vi "Waveform and Laser Controls V6.vi"() -> ()   [LabVIEW 2016]
uses:
  <vilib>/rvi/DataTransferAndStorage/Container/XNode/niFpgaContainer.xnode
  <vilib>/rvi/Memory/Memory_Emulation/nirvimemoryEmulation.vi
  <vilib>/rvi/Memory/Memory_Emulation/nirvimemoryFastEmulation.vi
  <vilib>/eio/EIONode/EIONode.xnode
  <vilib>/rvi/eio/common/nirviEmuTemplateMethod_errors.vi
  <vilib>/Platform/TimedLoop/XDataNode/wakeup.ctl
  <vilib>/Platform/TimedLoop/XDataNode/XDNodeRunTimeDep.lvlib
  <vilib>/Platform/TimedLoop/XDataNode/nitl_modes.ctl
  <vilib>/Platform/TimedLoop/XDataNode/timing_clust.ctl
  <vilib>/Platform/TimedLoop/XDataNode/XDataNode.xnode
  Waveform Scan Parameters.ctl
panel:
  out "Image Done?":bool
  in  "775 AOM (I16)":i16=16500
  in  "590 Analog Voltage (I16)":i16
  out "Laser Blank Trigger":bool
  in  "Laser On Time (Ticks)":u8=8
  in  "Sequences":u8=4
  in  "Laser Delay (Ticks)":u8
  in  "Laser States":u32
  in  "Blanking Off/Manual":bool
  in  "Z Piezo Axis":i16
  in  "Y Piezo Axis":i16
  in  "X Piezo Axis":i16
  out "End Linear Ramp":bool
  in  "End of Linear Ramp":u32
  in  "Z Stack Start Position (I16)":i16
  in  "Frames Per Z Step":u8
  in  "Number of Z Steps":u8
  in  "Z Step Size (I16)":i16
  in  "Stop Sync Signal":bool
  in  "Accums Per Line":u32[](array[numeric])=[0, 0, 0, 0]
  in  "Number of Lines":u32
  out "Frame Trigger":bool
  in  "Reset Position Error":bool
  in  "Galvo 1 Position (I16)":i16
  in  "Galvo 2 Position (I16)":i16
  in  "WF 3 Data Loaded":bool
  in  "WF 2 Data Loaded":bool
  in  "Waveform Scan Parameters":T1={"Scanning Mode"=0, "Fast Axis WF Length (Elements)"=0, "Fast Axis Sample Period (Ticks)"=40, "Slow Axis 1 WF Length (Elements)"=0, "Slow Axis 1 Sample Period (Ticks)"=40, "Slow Axis 1 Delay (25 ns) Steps"=40, "Slow Axis 2 WFLength (Elements)"=0, "Slow Axis 2 Sample Period (Ticks)"=40, "Slow Axis 2 Delay (25 ns) Steps"=40}
  in  "Resonant Mirror":T2
  in  "Galvo Mirror 2":T3
  in  "Galvo Mirror 1":T3
  in  "Start Waveforms":bool
  in  "Unused Axis Offset":i16
  in  "Slow Axis 2 Waveform Element":i16
  in  "Fast Axis Waveform Element":i16
  in  "Slow Axis 1 Waveform Element":i16
  in  "WF 1 Data Loaded":bool
  # "Copyright (C) 2020 Edward S Allgeyer\n\nRedistribution and use in source and binary forms, with or without\nmodification, are permitted provided that the following conditions\nare met:\n\n1. Redistributions of source code must retain the above copyright\n   notice, this list of conditions and the following disclaimer.\n\n2. Redistributions in binary form must reproduce the above copyright\n   notice, this list of conditions and the following disclaimer in\n   the documentation and/or other materials provided with the\n   distribution.\n\n3. Neither the name of the copyright holder nor the names of its\n   contributors may be used to endorse or promote products derived\n   from this software without specific prior written permission.\n\nTHIS SOFTWARE IS PROVIDED BY THE COPYRIGHT HOLDERS AND CONTRIBUTORS\n\"AS IS\" AND ANY EXPRESS OR IMPLIED WARRANTIES, INCLUDING, BUT NOT\nLIMITED TO, THE IMPLIED WARRANTIES OF MERCHANTABILITY AND FITNESS\nFOR A PARTICULAR PURPOSE ARE DISCLAIMED. IN NO EVENT SHALL THE\nCOPYRIGHT HOLDER OR CONTRIBUTORS BE LIABLE FOR ANY DIRECT, INDIRECT,\nINCIDENTAL, SPECIAL, EXEMPLARY, OR CONSEQUENTIAL DAMAGES (INCLUDING,\nBUT NOT LIMITED TO, PROCUREMENT OF SUBSTITUTE GOODS OR SERVICES;\nLOSS OF USE, DATA, OR PROFITS; OR BUSINESS INTERRUPTION) HOWEVER\nCAUSED AND ON ANY THEORY OF LIABILITY, WHETHER IN CONTRACT, STRICT\nLIABILITY, OR TORT (INCLUDING NEGLIGENCE OR OTHERWISE) ARISING IN\nANY WAY OUT OF THE USE OF THIS SOFTWARE, EVEN IF ADVISED OF THE\nPOSSIBILITY OF SUCH DAMAGE."
  # "V2 - Adding in a line clock\nV3 - Cluster Scan Parameters"
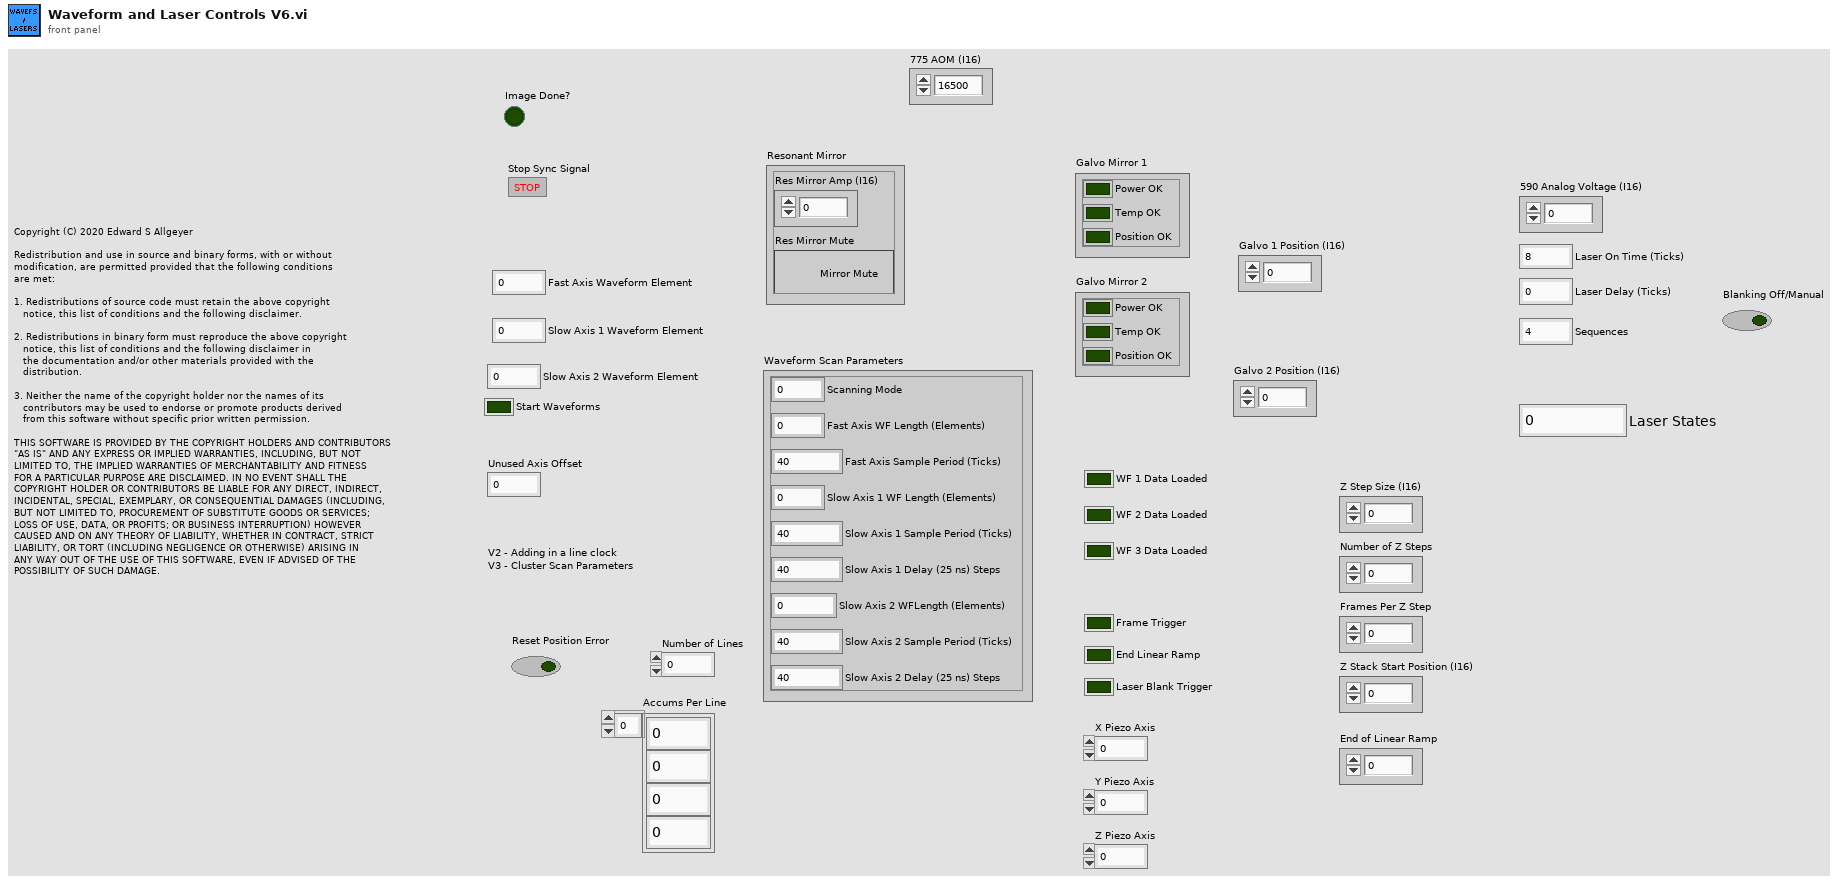
[diagram p1: front panel]
types:
  T1 = typedef "Waveform Scan Parameters.ctl" = cluster{"Scanning Mode":u8, "Fast Axis WF Length (Elements)":i32, "Fast Axis Sample Period (Ticks)":u32, "Slow Axis 1 WF Length (Elements)":i32, "Slow Axis 1 Sample Period (Ticks)":u32, "Slow Axis 1 Delay (25 ns) Steps":i32, "Slow Axis 2 WFLength (Elements)":i32, "Slow Axis 2 Sample Period (Ticks)":u32, "Slow Axis 2 Delay (25 ns) Steps":i32}
  T2 = cluster{"Res Mirror Amp (I16)":i16, "Res Mirror Mute":bool}
  T3 = cluster{"Power OK":bool, "Temp OK":bool, "Position OK":bool}
  T4 = typedef "XDNodeRunTimeDep.lvlib/timing_clust.ctl" = cluster{"Expected End [f-1]":u64, "Actual End [f-1]":u64, "Finished Late? [f-1]":bool, "Expected End [i-1]":u64, "Actual End [i-1]":u64, "Finished Late? [i-1]":bool, "Expected Start [i]":u64, "Actual Start [i]":u64, "Expected Start [f]":u64, "Actual Start [f]":u64, "Source Name":string, "Structure Name":string, "Period":i64, "Deadline":i64, "Offset":i64, "Start":i64, "Priority":i32, "Timeout":i32, "Mode":T5, "Wakeup Reason":T6, "Error":errorcluster, "Source Type":string, "Secondary Source Type":string, "Global End Time":u64, "Global Start Time":u64, "Frame Duration":u64, "Iteration Duration":u64, "Assigned CPU":i32, "I/O Scan Engine Mode":u32}
  T5 = typedef "XDNodeRunTimeDep.lvlib/nitl_modes.ctl" = enum32{"No Change", "Process missed periods, maintain original phase", "Discard missed periods, maintain original phase", "Process missed periods, ignore original phase", "Discard missed periods, ignore original phase"}
  T6 = typedef "XDNodeRunTimeDep.lvlib/wakeup.ctl" = enum32{"Normal", "Aborted", "Asynchronous wakeup", "Timing source error", "Timed loop error", "Timeout"}
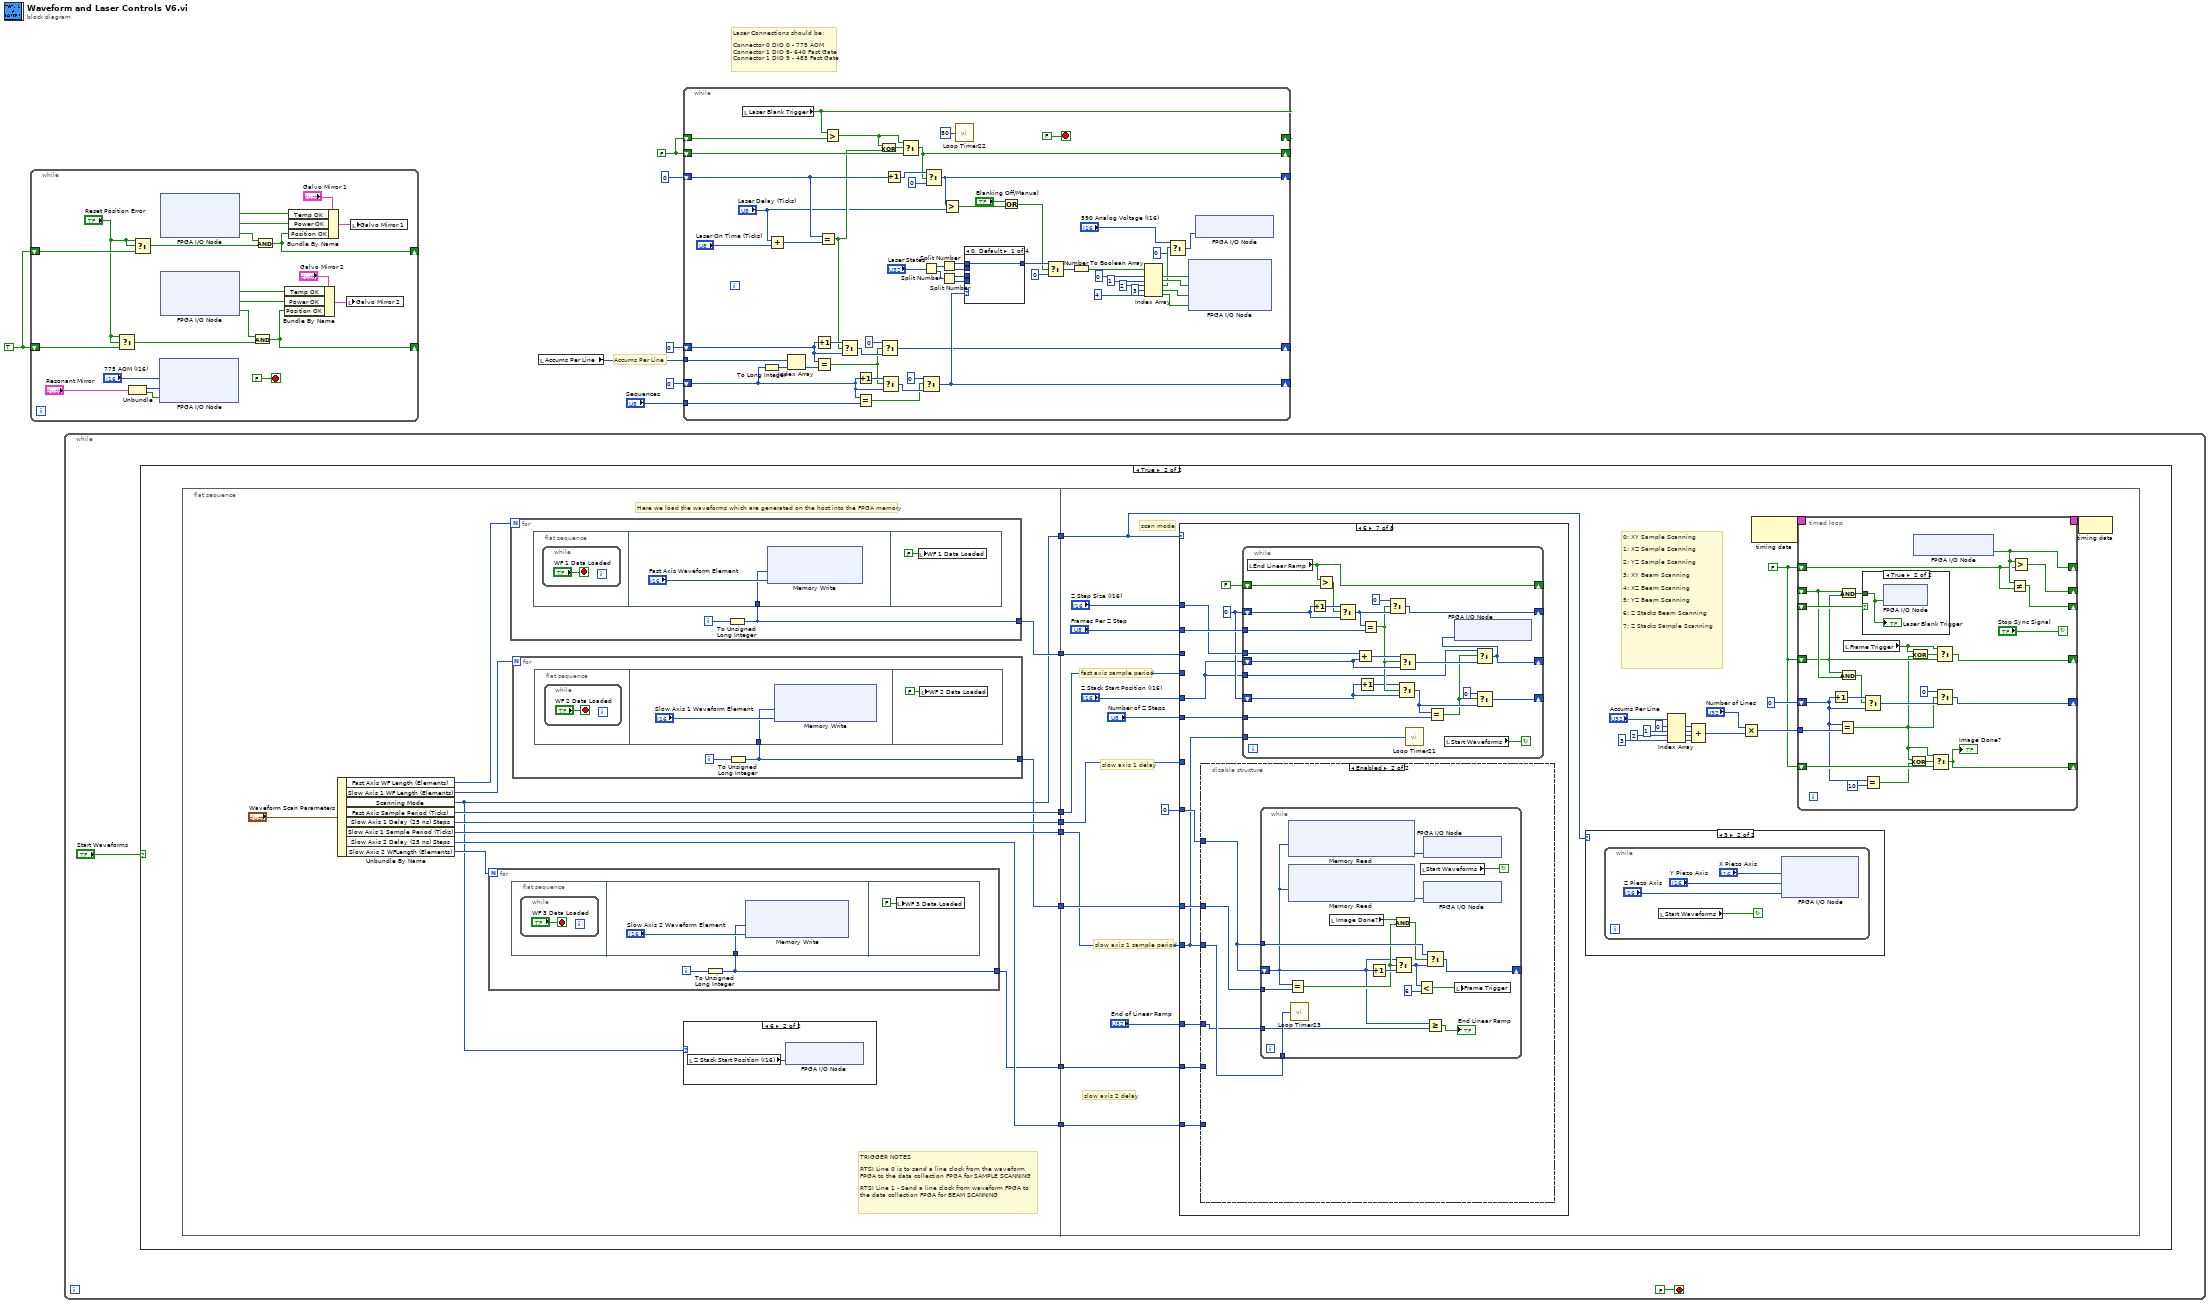
[diagram p0: block diagram]
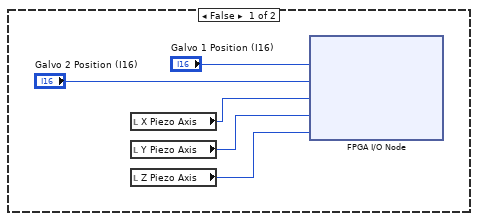
[diagram p5: hidden frame]
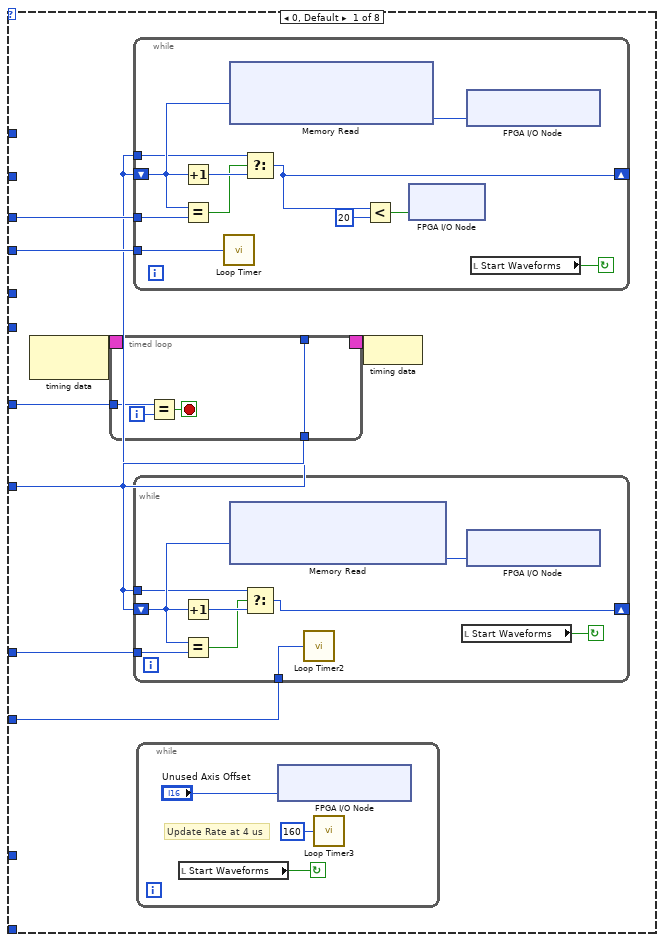
[diagram p9: hidden frame]
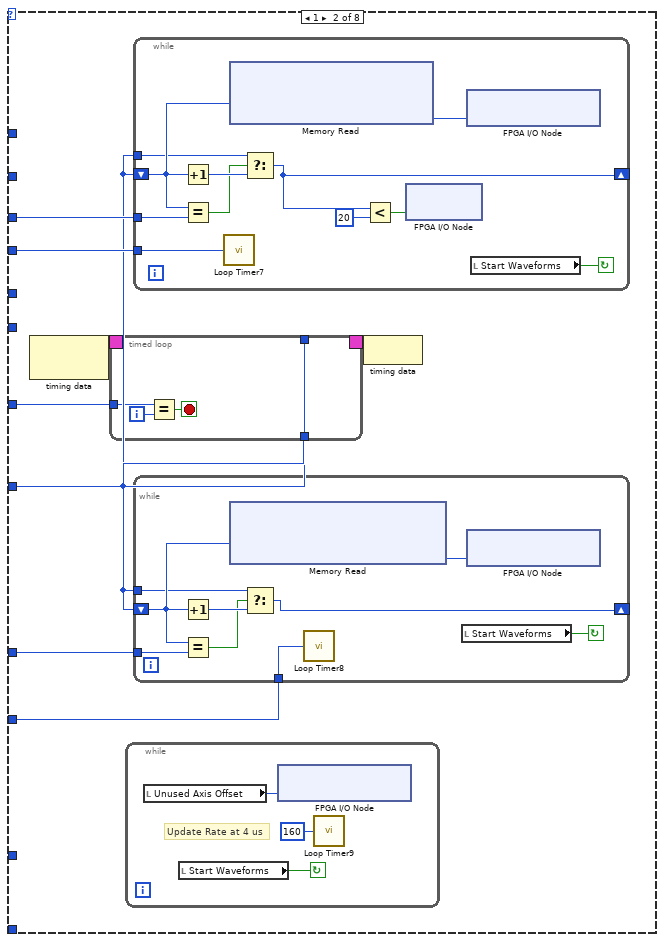
[diagram p10: hidden frame]
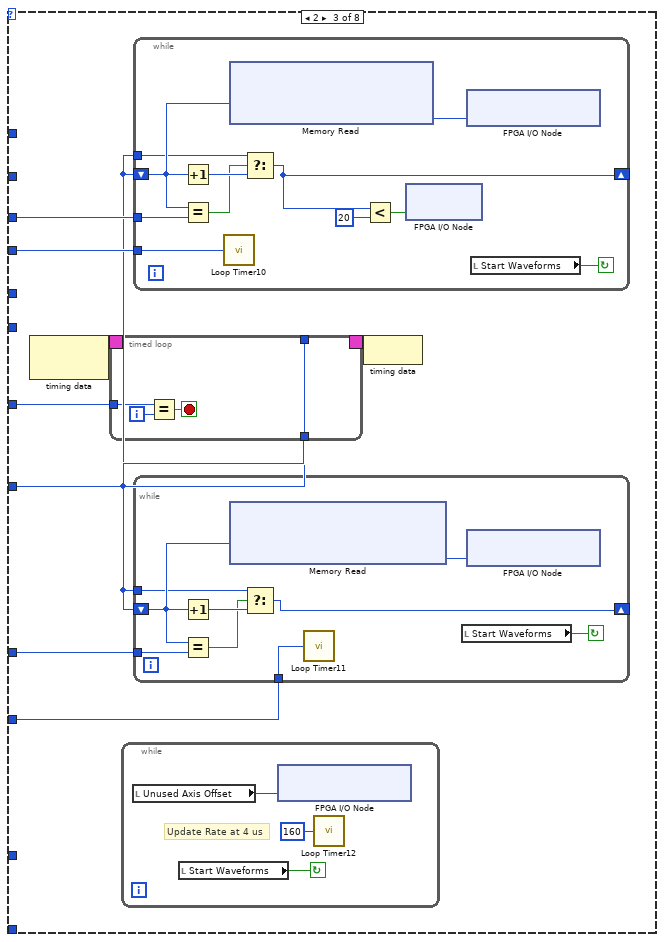
[diagram p11: hidden frame]
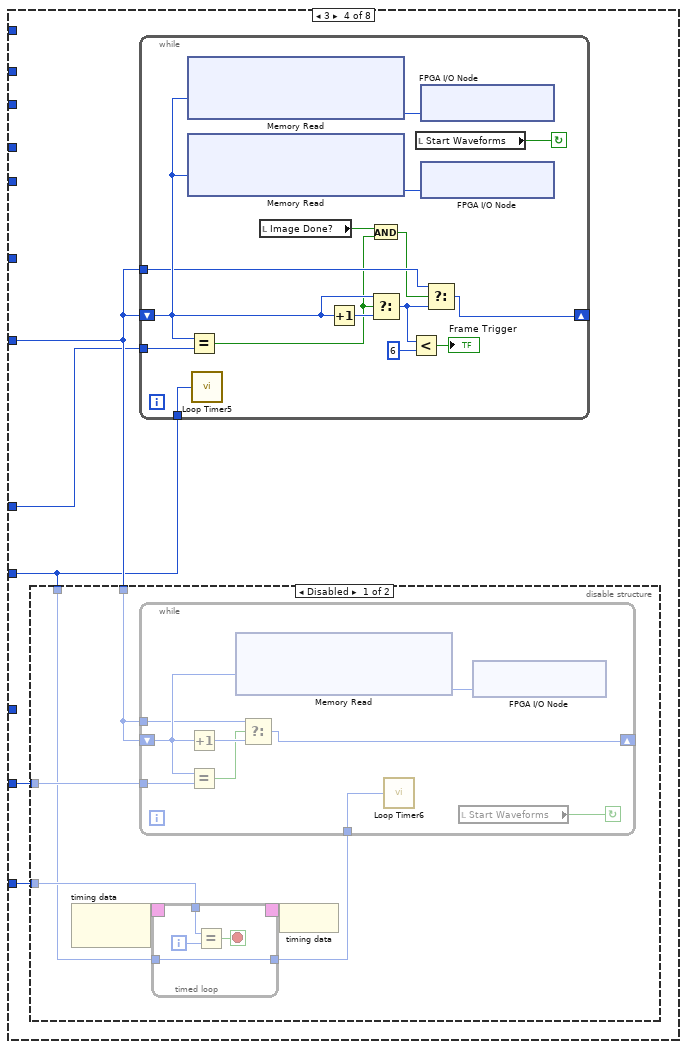
[diagram p12: hidden frame]
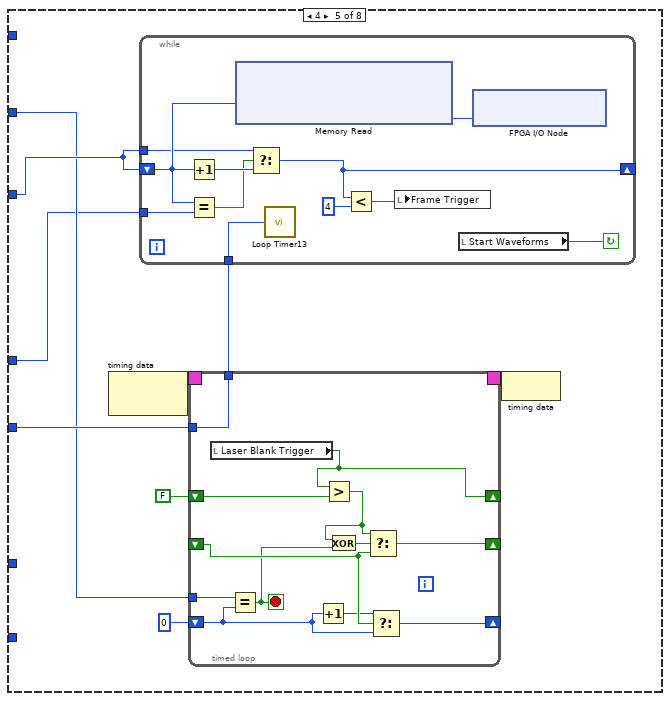
[diagram p14: hidden frame]
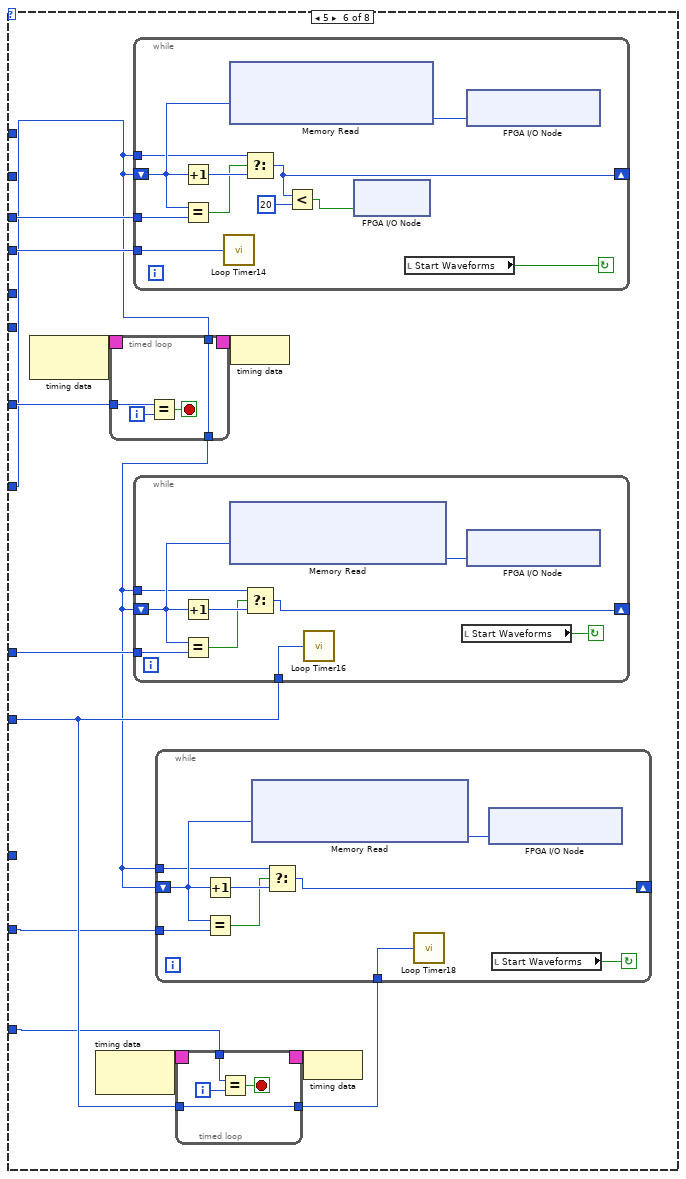
[diagram p15: hidden frame]
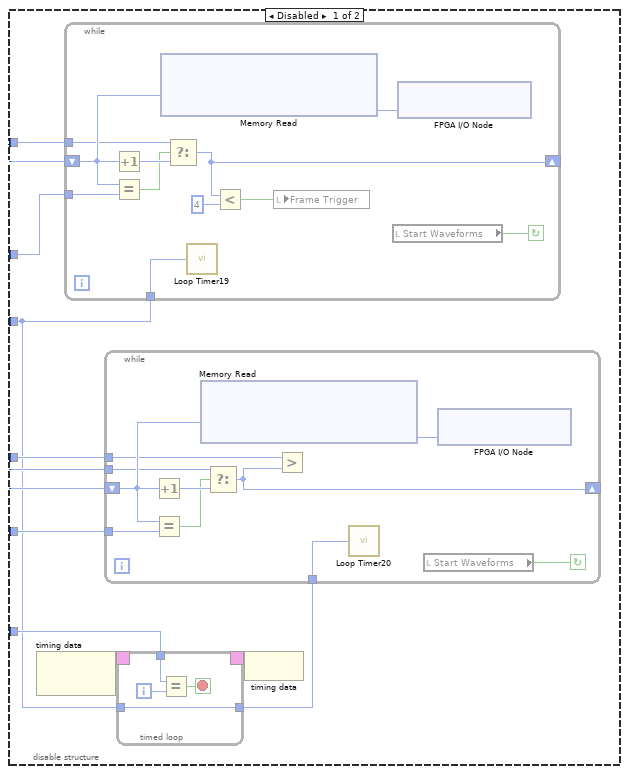
[diagram p16: hidden frame]
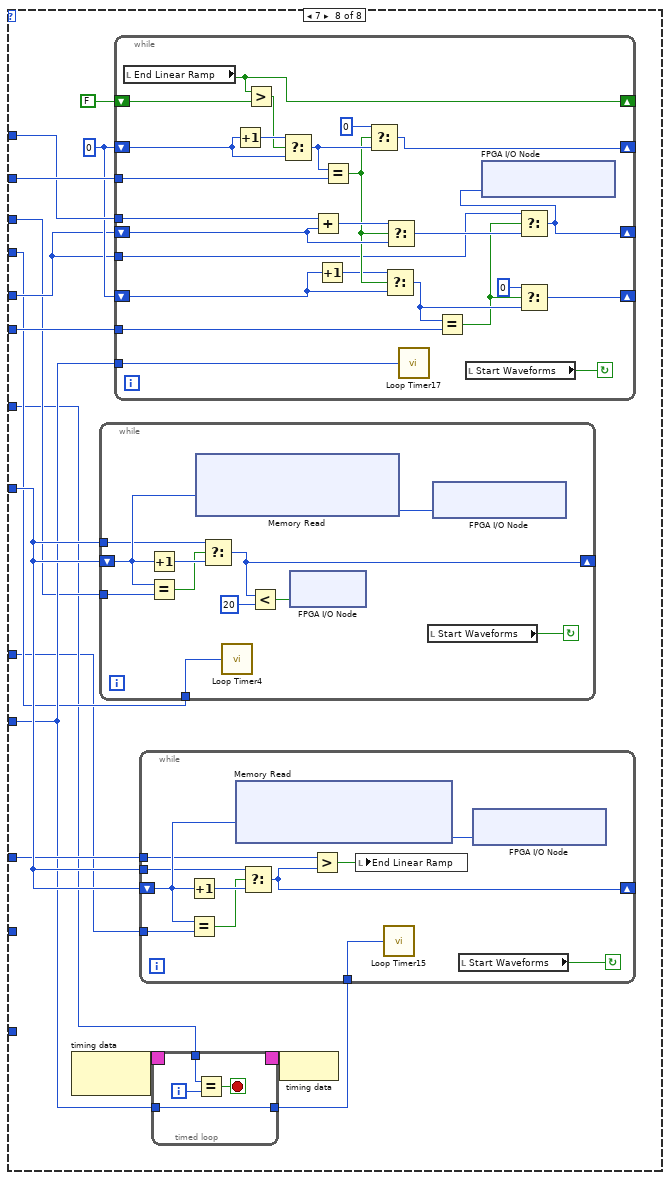
[diagram p17: hidden frame]
diagram:
  w2 = FALSE
  w7 = TRUE
  # "Laser Connections should be:\n\nConnector 0 DIO 0 - 775 AOM\nConnector 1 DIO 8- 640 Fast Gate\nConnector 1 DIO 9 - 485 Fast Gate"
  # "Accums Per Line"
  n1 = while {
    shift-right: [w14] -> _
    shift-left: w7 -> [w16]
    shift-right: [w10] -> _
    shift-left: w7 -> [w12]
    stop <- FALSE stop-if-true
    n2 = Select(t="Reset Position Error", s="Reset Position Error", f=w16) -> (s? t:f=w15:bool)
    n3 = Unbundle("Resonant Mirror") -> ("Res Mirror Amp (I16)"=w27:i16, "Res Mirror Mute"=w26:bool)
    n4 = Select(t="Reset Position Error", s="Reset Position Error", f=w12) -> (s? t:f=w11:bool)
    n5 = xnode "FPGA I/O Node"("Connector0/AO4"="775 AOM (I16)", "Connector0/AO7"=w27, "Connector0/DIO7"=w26) -> ()  [unwired: 4 in, 4 out]
    n6 = xnode "FPGA I/O Node"() -> ("Connector0/DIO1"=w25:bool, "Connector0/DIO2"=w24:bool, "Connector0/DIO3"=w13:bool)  [unwired: 4 in, 4 out]
    n7 = xnode "FPGA I/O Node"() -> ("Connector0/DIO4"=w18:bool, "Connector0/DIO5"=w19:bool, "Connector0/DIO6"=w17:bool)  [unwired: 4 in, 4 out]
    n8 = And(x=w17, y=w15) -> (x .and. y?=w14:bool)
    n9 = And(x=w13, y=w11) -> (x .and. y?=w10:bool)
    n10 = Bundle By Name(cluster="Galvo Mirror 2", "Temp OK"=w18, "Power OK"=w19, "Position OK"=w14) -> (w21:T3)
    n11 = Bundle By Name(cluster="Galvo Mirror 1", "Temp OK"=w25, "Power OK"=w24, "Position OK"=w10) -> (w23:T3)
    n12 = local write "Galvo Mirror 2"(w21) -> ()
    n13 = local write "Galvo Mirror 1"(w23) -> ()
  }
  n14 = while {
    stop <- FALSE stop-if-true
    n15 = case shown="True" "Start Waveforms" {
      frame False {
        n16 = local read "X Piezo Axis"() -> (w34:i16)
        n17 = local read "Y Piezo Axis"() -> (w33:i16)
        n18 = local read "Z Piezo Axis"() -> (w32:i16)
        n19 = xnode "FPGA I/O Node"("Connector0/AO5"="Galvo 1 Position (I16)", "Connector0/AO6"="Galvo 2 Position (I16)", "Connector0/AO1"=w34, "Connector0/AO2"=w33, "Connector0/AO3"=w32) -> ()  [unwired: 5 in, 5 out]
      }
      frame True {
        n20 = flat-sequence {
          tunnel: [w56] -> w44
          tunnel: [w46] -> w43
          tunnel: [w47] -> w42
          tunnel: [w45] -> w41
          tunnel: [w54] -> w40
          tunnel: [w53] -> w39
          tunnel: [w52] -> w38
          tunnel: [w51] -> w37
          tunnel: w44 -> [w105]
          tunnel: w43 -> [w104]
          tunnel: w42 -> [w102]
          tunnel: w41 -> [w78]
          tunnel: w40 -> [w101]
          tunnel: w39 -> [w100]
          tunnel: w38 -> [w99]
          tunnel: w37 -> [w98]
          frame #0 {
            # "TRIGGER NOTES\n\nRTSI Line 0 is to send a line clock from the waveform\nFPGA to the data collection FPGA for SAMPLE SCANNING\n\nRTSI Line 1 - Send a line clock from waveform FPGA to\nthe data collection FPGA for BEAM SCANNING"
            # "Here we load the waveforms which are generated on the host into the FPGA memory"
            n21 = Unbundle By Name("Waveform Scan Parameters") -> ("Fast Axis WF Length (Elements)"=w50:i32, "Slow Axis 1 WF Length (Elements)"=w49:i32, "Scanning Mode"=w45:u8, "Fast Axis Sample Period (Ticks)"=w54:u32, "Slow Axis 1 Delay (25 ns) Steps"=w53:i32, "Slow Axis 1 Sample Period (Ticks)"=w52:u32, "Slow Axis 2 Delay (25 ns) Steps"=w51:i32, "Slow Axis 2 WFLength (Elements)"=w48:i32)
            n22 = for {
              N: w48 -> [_]
              tunnel: [w58] -> w46
              i -> [w59]
              n23 = flat-sequence {
                tunnel: w58 -> [w61]
                frame #0 {
                  n24 = while {
                    stop <- "WF 3 Data Loaded" stop-if-true
                  }
                }
                frame #1 {
                  n25 = xnode ("Memory Write")("Address"=w61, "Data"="Slow Axis 2 Waveform Element") -> ()  [unwired: 1 in, 1 out]
                }
                frame #2 {
                  n26 = local write "WF 3 Data Loaded"(FALSE ("Host Data Loaded")) -> ()
                }
              }
              n27 = To Unsigned Long Integer(number=w59) -> (unsigned 32bit integer=w58:u32)
            }
            n28 = for {
              N: w50 -> [_]
              tunnel: [w70] -> w56
              i -> [w71]
              n29 = flat-sequence {
                tunnel: w70 -> [w73]
                frame #0 {
                  n30 = while {
                    stop <- "WF 1 Data Loaded" stop-if-true
                  }
                }
                frame #1 {
                  n31 = xnode ("Memory Write")("Address"=w73, "Data"="Fast Axis Waveform Element") -> ()  [unwired: 1 in, 1 out]
                }
                frame #2 {
                  n32 = local write "WF 1 Data Loaded"(FALSE ("Host Data Loaded")) -> ()
                }
              }
              n33 = To Unsigned Long Integer(number=w71) -> (unsigned 32bit integer=w70:u32)
            }
            n34 = for {
              N: w49 -> [_]
              tunnel: [w64] -> w47
              i -> [w65]
              n35 = flat-sequence {
                tunnel: w64 -> [w67]
                frame #0 {
                  n36 = while {
                    stop <- "WF 2 Data Loaded" stop-if-true
                  }
                }
                frame #1 {
                  n37 = xnode ("Memory Write")("Address"=w67, "Data"="Slow Axis 1 Waveform Element") -> ()  [unwired: 1 in, 1 out]
                }
                frame #2 {
                  n38 = local write "WF 2 Data Loaded"(FALSE ("Host Data Loaded")) -> ()
                }
              }
              n39 = To Unsigned Long Integer(number=w65) -> (unsigned 32bit integer=w64:u32)
            }
            n40 = case shown="6" w45 {
              frame 0, Default {
              }
              frame 6 {
                n41 = local read "Z Stack Start Position (I16)"() -> (w57:i16)
                n42 = xnode "FPGA I/O Node"("Connector0/AO3"=w57) -> ()  [unwired: 1 in, 1 out]
              }
            }
          }
          frame #1 {
            w76 = FALSE
            # "slow axis 2 delay"
            # "slow axis 1 sample period"
            # "slow axis 1 delay"
            # "fast axis sample period"
            # "scan mode"
            # "0: XY Sample Scanning\n\n1: XZ Sample Scanning\n\n2: YZ Sample Scanning\n\n3: XY Beam Scanning\n\n4: XZ Beam Scanning\n\n5: YZ Beam Scanning\n\n6: Z Stacks Beam Scanning\n\n7: Z Stacks Sample Scanning"
            n43 = case shown="6" w78 {
              tunnel: w105 -> [w146 w186 w226 _ _ w353 _ w497]
              tunnel: w101 -> [w145 w185 w225 _ _ w352 _ w498]
              tunnel: w104 -> [_ _ _ w264 _ w347 w410 _]
              tunnel: u32 0 -> [w140 w180 w220 w263 w312 w349 w409 w510]
              tunnel: w100 -> [w144 w184 w224 _ w310 w351 _ w496]
              tunnel: w98 -> [_ _ _ w262 _ w346 w408 _]
              tunnel: w102 -> [w142 w182 w222 w260 w309 w350 w407 w495]
              tunnel: w99 -> [w141 w181 w221 w261 w311 w348 w399 w499]
              tunnel: "Frames Per Z Step" -> [_ _ _ _ _ _ w405 w506]
              tunnel: "Z Stack Start Position (I16)" -> [_ _ _ _ _ _ w401 w502]
              tunnel: "Z Step Size (I16)" -> [_ _ _ _ _ _ w404 w505]
              tunnel: "Number of Z Steps" -> [_ _ _ _ _ _ w402 w503]
              tunnel: "End of Linear Ramp" -> [_ _ _ _ _ _ w400 w501]
              frame 0, Default {
                n44 = node-c288() -> (w148:T4)  [unwired: 1 in]
                n45 = timed-loop {
                  timing: w148 -> [_]
                  timing-out: [_] -> w147
                  tunnel: w144 -> [w153]
                  tunnel: w140 -> [w152]
                  tunnel: [w152] -> w143
                  i -> [w155]
                  stop <- w154 stop-if-true
                  n46 = Equal?(x=w153, y=w155) -> (x = y?=w154:bool)
                }
                n47 = while {
                  shift-right: [w171] -> _
                  shift-left: w140 -> [w177]
                  tunnel: w146 -> [w178]
                  tunnel: w145 -> [w175]
                  tunnel: w140 -> [w174]
                  stop <- w173 continue-if-true
                  n48 = Increment(x=w177) -> (x+1=w179:u32)
                  n49 = Equal?(x=w177, y=w178) -> (x = y?=w172:bool)
                  n50 = call "Loop Timer"("Count(Ticks)"=w175) -> ()  [unwired: 1 out]
                  n51 = xnode ("Memory Read")("Address"=w177) -> ("Data"=w176:i16)  [unwired: 1 in, 1 out]
                  n52 = Select(t=w174, s=w172, f=w179) -> (s? t:f=w171:u32)
                  n53 = Less?(x=w171, y=u32 20) -> (x < y?=w169:bool)
                  n54 = xnode "FPGA I/O Node"("TRIG0"=w169) -> ()  [unwired: 1 in, 1 out]
                  n55 = xnode "FPGA I/O Node"("Connector0/AO1"=w176) -> ()  [unwired: 1 in, 1 out]
                  n56 = local read "Start Waveforms"() -> (w173:bool)
                }
                n57 = while {
                  shift-right: [w167] -> _
                  shift-left: w143 -> [w164]
                  tunnel: w142 -> [w166]
                  tunnel: w143 -> [w162]
                  tunnel: w141 -> [w161]
                  stop <- w160 continue-if-true
                  n58 = Increment(x=w164) -> (x+1=w168:u32)
                  n59 = Equal?(x=w164, y=w166) -> (x = y?=w165:bool)
                  n60 = xnode ("Memory Read")("Address"=w164) -> ("Data"=w163:i16)  [unwired: 1 in, 1 out]
                  n61 = Select(t=w162, s=w165, f=w168) -> (s? t:f=w167:u32)
                  n62 = call "Loop Timer2"("Count(Ticks)"=w161) -> ()  [unwired: 1 out]
                  n63 = local read "Start Waveforms"() -> (w160:bool)
                  n64 = xnode "FPGA I/O Node"("Connector0/AO2"=w163) -> ()  [unwired: 1 in, 1 out]
                }
                n65 = while {
                  stop <- w149 continue-if-true
                  # "Update Rate at 4 us"
                  n66 = local read "Start Waveforms"() -> (w149:bool)
                  n67 = xnode "FPGA I/O Node"("Connector0/AO3"="Unused Axis Offset") -> ()  [unwired: 1 in, 1 out]
                  n68 = call "Loop Timer3"("Count(Ticks)"=u32 160) -> ()  [unwired: 1 out]
                }
                n69 = node-c288(w147) -> ()
              }
              frame 1 {
                n70 = node-c288() -> (w188:T4)  [unwired: 1 in]
                n71 = timed-loop {
                  timing: w188 -> [_]
                  timing-out: [_] -> w187
                  tunnel: w184 -> [w193]
                  tunnel: w180 -> [w192]
                  tunnel: [w192] -> w183
                  i -> [w195]
                  stop <- w194 stop-if-true
                  n72 = Equal?(x=w193, y=w195) -> (x = y?=w194:bool)
                }
                n73 = while {
                  stop <- w190 continue-if-true
                  # "Update Rate at 4 us"
                  n74 = local read "Unused Axis Offset"() -> (w189:i16)
                  n75 = local read "Start Waveforms"() -> (w190:bool)
                  n76 = xnode "FPGA I/O Node"("Connector0/AO2"=w189) -> ()  [unwired: 1 in, 1 out]
                  n77 = call "Loop Timer9"("Count(Ticks)"=u32 160) -> ()  [unwired: 1 out]
                }
                n78 = while {
                  shift-right: [w211] -> _
                  shift-left: w180 -> [w217]
                  tunnel: w186 -> [w218]
                  tunnel: w185 -> [w215]
                  tunnel: w180 -> [w214]
                  stop <- w213 continue-if-true
                  n79 = Increment(x=w217) -> (x+1=w219:u32)
                  n80 = Equal?(x=w217, y=w218) -> (x = y?=w212:bool)
                  n81 = call "Loop Timer7"("Count(Ticks)"=w215) -> ()  [unwired: 1 out]
                  n82 = xnode ("Memory Read")("Address"=w217) -> ("Data"=w216:i16)  [unwired: 1 in, 1 out]
                  n83 = Select(t=w214, s=w212, f=w219) -> (s? t:f=w211:u32)
                  n84 = Less?(x=w211, y=u32 20) -> (x < y?=w209:bool)
                  n85 = xnode "FPGA I/O Node"("TRIG0"=w209) -> ()  [unwired: 1 in, 1 out]
                  n86 = xnode "FPGA I/O Node"("Connector0/AO1"=w216) -> ()  [unwired: 1 in, 1 out]
                  n87 = local read "Start Waveforms"() -> (w213:bool)
                }
                n88 = while {
                  shift-right: [w207] -> _
                  shift-left: w183 -> [w204]
                  tunnel: w182 -> [w206]
                  tunnel: w183 -> [w202]
                  tunnel: w181 -> [w201]
                  stop <- w200 continue-if-true
                  n89 = Increment(x=w204) -> (x+1=w208:u32)
                  n90 = Equal?(x=w204, y=w206) -> (x = y?=w205:bool)
                  n91 = xnode ("Memory Read")("Address"=w204) -> ("Data"=w203:i16)  [unwired: 1 in, 1 out]
                  n92 = Select(t=w202, s=w205, f=w208) -> (s? t:f=w207:u32)
                  n93 = call "Loop Timer8"("Count(Ticks)"=w201) -> ()  [unwired: 1 out]
                  n94 = local read "Start Waveforms"() -> (w200:bool)
                  n95 = xnode "FPGA I/O Node"("Connector0/AO3"=w203) -> ()  [unwired: 1 in, 1 out]
                }
                n96 = node-c288(w187) -> ()
              }
              frame 2 {
                n97 = node-c288() -> (w228:T4)  [unwired: 1 in]
                n98 = timed-loop {
                  timing: w228 -> [_]
                  timing-out: [_] -> w227
                  tunnel: w224 -> [w233]
                  tunnel: w220 -> [w232]
                  tunnel: [w232] -> w223
                  i -> [w235]
                  stop <- w234 stop-if-true
                  n99 = Equal?(x=w233, y=w235) -> (x = y?=w234:bool)
                }
                n100 = while {
                  stop <- w230 continue-if-true
                  # "Update Rate at 4 us"
                  n101 = local read "Unused Axis Offset"() -> (w229:i16)
                  n102 = local read "Start Waveforms"() -> (w230:bool)
                  n103 = xnode "FPGA I/O Node"("Connector0/AO1"=w229) -> ()  [unwired: 1 in, 1 out]
                  n104 = call "Loop Timer12"("Count(Ticks)"=u32 160) -> ()  [unwired: 1 out]
                }
                n105 = while {
                  shift-right: [w251] -> _
                  shift-left: w220 -> [w257]
                  tunnel: w226 -> [w258]
                  tunnel: w225 -> [w255]
                  tunnel: w220 -> [w254]
                  stop <- w253 continue-if-true
                  n106 = Increment(x=w257) -> (x+1=w259:u32)
                  n107 = Equal?(x=w257, y=w258) -> (x = y?=w252:bool)
                  n108 = call "Loop Timer10"("Count(Ticks)"=w255) -> ()  [unwired: 1 out]
                  n109 = xnode ("Memory Read")("Address"=w257) -> ("Data"=w256:i16)  [unwired: 1 in, 1 out]
                  n110 = Select(t=w254, s=w252, f=w259) -> (s? t:f=w251:u32)
                  n111 = Less?(x=w251, y=u32 20) -> (x < y?=w249:bool)
                  n112 = xnode "FPGA I/O Node"("TRIG0"=w249) -> ()  [unwired: 1 in, 1 out]
                  n113 = xnode "FPGA I/O Node"("Connector0/AO2"=w256) -> ()  [unwired: 1 in, 1 out]
                  n114 = local read "Start Waveforms"() -> (w253:bool)
                }
                n115 = while {
                  shift-right: [w247] -> _
                  shift-left: w223 -> [w244]
                  tunnel: w222 -> [w246]
                  tunnel: w223 -> [w242]
                  tunnel: w221 -> [w241]
                  stop <- w240 continue-if-true
                  n116 = Increment(x=w244) -> (x+1=w248:u32)
                  n117 = Equal?(x=w244, y=w246) -> (x = y?=w245:bool)
                  n118 = xnode ("Memory Read")("Address"=w244) -> ("Data"=w243:i16)  [unwired: 1 in, 1 out]
                  n119 = Select(t=w242, s=w245, f=w248) -> (s? t:f=w247:u32)
                  n120 = call "Loop Timer11"("Count(Ticks)"=w241) -> ()  [unwired: 1 out]
                  n121 = local read "Start Waveforms"() -> (w240:bool)
                  n122 = xnode "FPGA I/O Node"("Connector0/AO3"=w243) -> ()  [unwired: 1 in, 1 out]
                }
                n123 = node-c288(w227) -> ()
              }
              frame 3 {
                n124 = disable-structure shown="Disabled" {
                  disable-tunnel: w264 -> [w269 _]
                  disable-tunnel: w263 -> [w268 _]
                  disable-tunnel: w262 -> [w267 _]
                  disable-tunnel: w261 -> [w265 _]
                  frame Disabled {
                    n125 = node-c288() -> (w271:T4)  [unwired: 1 in]
                    n126 = timed-loop {
                      timing: w271 -> [_]
                      timing-out: [_] -> w270
                      tunnel: w265 -> [w281]
                      tunnel: [w281] -> w266
                      tunnel: w267 -> [w282]
                      i -> [w284]
                      stop <- w283 stop-if-true
                      n127 = Equal?(x=w282, y=w284) -> (x = y?=w283:bool)
                    }
                    n128 = while {
                      shift-right: [w279] -> _
                      shift-left: w268 -> [w277]
                      tunnel: w269 -> [w278]
                      tunnel: w266 -> [w275]
                      tunnel: w268 -> [w274]
                      stop <- w273 continue-if-true
                      n129 = Increment(x=w277) -> (x+1=w280:u32)
                      n130 = Equal?(x=w277, y=w278) -> (x = y?=w272:bool)
                      n131 = xnode ("Memory Read")("Address"=w277) -> ("Data"=w276:i16)  [unwired: 1 in, 1 out]
                      n132 = Select(t=w274, s=w272, f=w280) -> (s? t:f=w279:u32)
                      n133 = call "Loop Timer6"("Count(Ticks)"=w275) -> ()  [unwired: 1 out]
                      n134 = local read "Start Waveforms"() -> (w273:bool)
                      n135 = xnode "FPGA I/O Node"("Connector0/AO6"=w276) -> ()  [unwired: 1 in, 1 out]
                    }
                    n136 = node-c288(w270) -> ()
                  }
                  frame Enabled {
                  }
                }
                n137 = while {
                  shift-right: [w293] -> _
                  shift-left: w263 -> [w295]
                  tunnel: w260 -> [w302]
                  tunnel: w261 -> [w300]
                  tunnel: w263 -> [w292]
                  stop <- w299 continue-if-true
                  n138 = xnode ("Memory Read")("Address"=w295) -> ("Data"=w296:i16)  [unwired: 1 in, 1 out]
                  n139 = xnode ("Memory Read")("Address"=w295) -> ("Data"=w301:i16)  [unwired: 1 in, 1 out]
                  n140 = Equal?(x=w295, y=w302) -> (x = y?=w291:bool)
                  n141 = call "Loop Timer5"("Count(Ticks)"=w300) -> ()  [unwired: 1 out]
                  n142 = local read "Image Done?"() -> (w290:bool)
                  n143 = Increment(x=w295) -> (x+1=w303:u32)
                  n144 = And(x=w290, y=w291) -> (x .and. y?=w289:bool)
                  n145 = Select(t=w295, s=w291, f=w303) -> (s? t:f=w294:u32)
                  n146 = Less?(x=w294, y=u32 6) -> (x < y?=→"Frame Trigger":bool)
                  n147 = local read "Start Waveforms"() -> (w299:bool)
                  n148 = xnode "FPGA I/O Node"("Connector0/AO6"=w296) -> ()  [unwired: 1 in, 1 out]
                  n149 = xnode "FPGA I/O Node"("Connector0/AO5"=w301) -> ()  [unwired: 1 in, 1 out]
                  n150 = Select(t=w292, s=w289, f=w294) -> (s? t:f=w293:u32)
                }
              }
              frame 4 {
                n151 = node-c288() -> (w308:T4)  [unwired: 1 in]
                n152 = timed-loop {
                  timing: w308 -> [_]
                  timing-out: [_] -> w307
                  tunnel: w311 -> [w315]
                  shift-right: [w313] -> _
                  shift-left: FALSE -> [w324]
                  shift-right: [w321] -> _
                  shift-left: _ -> [w320]
                  shift-right: [w318] -> _
                  shift-left: 0 -> [w316]
                  tunnel: w310 -> [w317]
                  tunnel: [w315] -> w304
                  stop <- w314 stop-if-true
                  n153 = local read "Laser Blank Trigger"() -> (w313:bool)
                  n154 = Equal?(x=w317, y=w316) -> (x = y?=w314:bool)
                  n155 = Increment(x=w316) -> (x+1=w319:i32)
                  n156 = Greater?(x=w313, y=w324) -> (0:w322:bool)
                  n157 = Exclusive Or(1:w314, 2:w322) -> (0:w323:bool)
                  n158 = Select(t=w322, s=w323, f=w320) -> (s? t:f=w321:bool)
                  n159 = Select(t=w319, s=w320, f=w316) -> (s? t:f=w318:i32)
                }
                n160 = while {
                  shift-right: [w330] -> _
                  shift-left: w312 -> [w336]
                  tunnel: w309 -> [w338]
                  tunnel: w304 -> [w334]
                  tunnel: w312 -> [w333]
                  stop <- w332 continue-if-true
                  n161 = Increment(x=w336) -> (x+1=w339:u32)
                  n162 = Equal?(x=w336, y=w338) -> (x = y?=w337:bool)
                  n163 = xnode ("Memory Read")("Address"=w336) -> ("Data"=w335:i16)  [unwired: 1 in, 1 out]
                  n164 = Select(t=w333, s=w337, f=w339) -> (s? t:f=w330:u32)
                  n165 = call "Loop Timer13"("Count(Ticks)"=w334) -> ()  [unwired: 1 out]
                  n166 = Less?(x=w330, y=u32 4) -> (x < y?=w329:bool)
                  n167 = local write "Frame Trigger"(w329) -> ()
                  n168 = local read "Start Waveforms"() -> (w332:bool)
                  n169 = xnode "FPGA I/O Node"("Connector0/AO3"=w335) -> ()  [unwired: 1 in, 1 out]
                }
                n170 = node-c288(w307) -> ()
              }
              frame 5 {
                n171 = node-c288() -> (w345:T4)  [unwired: 1 in]
                n172 = node-c288() -> (w343:T4)  [unwired: 1 in]
                n173 = timed-loop {
                  timing: w345 -> [_]
                  timing-out: [_] -> w344
                  tunnel: w351 -> [w372]
                  tunnel: w349 -> [w371]
                  tunnel: [w371] -> w340
                  i -> [w374]
                  stop <- w373 stop-if-true
                  n174 = Equal?(x=w372, y=w374) -> (x = y?=w373:bool)
                }
                n175 = while {
                  shift-right: [w391] -> _
                  shift-left: w349 -> [w396]
                  tunnel: w353 -> [w397]
                  tunnel: w352 -> [w394]
                  tunnel: w349 -> [w393]
                  stop <- w389 continue-if-true
                  n176 = Increment(x=w396) -> (x+1=w398:u32)
                  n177 = Equal?(x=w396, y=w397) -> (x = y?=w392:bool)
                  n178 = call "Loop Timer14"("Count(Ticks)"=w394) -> ()  [unwired: 1 out]
                  n179 = xnode ("Memory Read")("Address"=w396) -> ("Data"=w395:i16)  [unwired: 1 in, 1 out]
                  n180 = Select(t=w393, s=w392, f=w398) -> (s? t:f=w391:u32)
                  n181 = Less?(x=w391, y=u32 20) -> (x < y?=w388:bool)
                  n182 = xnode "FPGA I/O Node"("TRIG0"=w388) -> ()  [unwired: 1 in, 1 out]
                  n183 = local read "Start Waveforms"() -> (w389:bool)
                  n184 = xnode "FPGA I/O Node"("Connector0/AO5"=w395) -> ()  [unwired: 1 in, 1 out]
                }
                n185 = while {
                  shift-right: [w386] -> _
                  shift-left: w340 -> [w383]
                  tunnel: w350 -> [w385]
                  tunnel: w340 -> [w381]
                  tunnel: w348 -> [w380]
                  stop <- w379 continue-if-true
                  n186 = Increment(x=w383) -> (x+1=w387:u32)
                  n187 = Equal?(x=w383, y=w385) -> (x = y?=w384:bool)
                  n188 = xnode ("Memory Read")("Address"=w383) -> ("Data"=w382:i16)  [unwired: 1 in, 1 out]
                  n189 = Select(t=w381, s=w384, f=w387) -> (s? t:f=w386:u32)
                  n190 = call "Loop Timer16"("Count(Ticks)"=w380) -> ()  [unwired: 1 out]
                  n191 = local read "Start Waveforms"() -> (w379:bool)
                  n192 = xnode "FPGA I/O Node"("Connector0/AO6"=w382) -> ()  [unwired: 1 in, 1 out]
                }
                n193 = timed-loop {
                  timing: w343 -> [_]
                  timing-out: [_] -> w342
                  tunnel: w348 -> [w363]
                  tunnel: [w363] -> w341
                  tunnel: w346 -> [w364]
                  i -> [w366]
                  stop <- w365 stop-if-true
                  n194 = Equal?(x=w364, y=w366) -> (x = y?=w365:bool)
                }
                n195 = while {
                  shift-right: [w361] -> _
                  shift-left: w340 -> [w358]
                  tunnel: w347 -> [w360]
                  tunnel: w341 -> [w356]
                  tunnel: w340 -> [w355]
                  stop <- w354 continue-if-true
                  n196 = Increment(x=w358) -> (x+1=w362:u32)
                  n197 = Equal?(x=w358, y=w360) -> (x = y?=w359:bool)
                  n198 = xnode ("Memory Read")("Address"=w358) -> ("Data"=w357:i16)  [unwired: 1 in, 1 out]
                  n199 = Select(t=w355, s=w359, f=w362) -> (s? t:f=w361:u32)
                  n200 = call "Loop Timer18"("Count(Ticks)"=w356) -> ()  [unwired: 1 out]
                  n201 = xnode "FPGA I/O Node"("Connector0/AO3"=w357) -> ()  [unwired: 1 in, 1 out]
                  n202 = local read "Start Waveforms"() -> (w354:bool)
                }
                n203 = node-c288(w344) -> ()
                n204 = node-c288(w342) -> ()
              }
              frame 6 {
                w403 = u8 0
                n205 = disable-structure shown="Enabled" {
                  disable-tunnel: w410 -> [w417 _]
                  disable-tunnel: w409 -> [w416 w451]
                  disable-tunnel: w408 -> [w415 _]
                  disable-tunnel: w407 -> [w414 w450]
                  disable-tunnel: w400 -> [w413 w449]
                  disable-tunnel: w399 -> [w411 w452]
                  frame Disabled {
                    n206 = node-c288() -> (w419:T4)  [unwired: 1 in]
                    n207 = while {
                      shift-right: [w440] -> _
                      shift-left: w416 -> [w446]
                      tunnel: w414 -> [w447]
                      tunnel: w411 -> [w444]
                      tunnel: w416 -> [w443]
                      stop <- w442 continue-if-true
                      n208 = Increment(x=w446) -> (x+1=w448:u32)
                      n209 = Equal?(x=w446, y=w447) -> (x = y?=w441:bool)
                      n210 = xnode ("Memory Read")("Address"=w446) -> ("Data"=w445:i16)  [unwired: 1 in, 1 out]
                      n211 = Select(t=w443, s=w441, f=w448) -> (s? t:f=w440:u32)
                      n212 = call "Loop Timer19"("Count(Ticks)"=w444) -> ()  [unwired: 1 out]
                      n213 = Less?(x=w440, y=u32 4) -> (x < y?=w438:bool)
                      n214 = local write "Frame Trigger"(w438) -> ()
                      n215 = local read "Start Waveforms"() -> (w442:bool)
                      n216 = xnode "FPGA I/O Node"("Connector0/AO5"=w445) -> ()  [unwired: 1 in, 1 out]
                    }
                    n217 = timed-loop {
                      timing: w419 -> [_]
                      timing-out: [_] -> w418
                      tunnel: w411 -> [w430]
                      tunnel: [w430] -> w412
                      tunnel: w415 -> [w431]
                      i -> [w433]
                      stop <- w432 stop-if-true
                      n218 = Equal?(x=w431, y=w433) -> (x = y?=w432:bool)
                    }
                    n219 = while {
                      shift-right: [w421] -> _
                      shift-left: w416 -> [w427]
                      tunnel: w417 -> [w428]
                      tunnel: w412 -> [w425]
                      tunnel: w416 -> [w424]
                      tunnel: w413 -> [w420]
                      stop <- w423 continue-if-true
                      n220 = Increment(x=w427) -> (x+1=w429:u32)
                      n221 = Equal?(x=w427, y=w428) -> (x = y?=w422:bool)
                      n222 = xnode ("Memory Read")("Address"=w427) -> ("Data"=w426:i16)  [unwired: 1 in, 1 out]
                      n223 = Select(t=w424, s=w422, f=w429) -> (s? t:f=w421:u32)
                      n224 = Greater?(x=w420, y=w421) -> ()  [unwired: 1 out]
                      n225 = call "Loop Timer20"("Count(Ticks)"=w425) -> ()  [unwired: 1 out]
                      n226 = local read "Start Waveforms"() -> (w423:bool)
                      n227 = xnode "FPGA I/O Node"("Connector0/AO6"=w426) -> ()  [unwired: 1 in, 1 out]
                    }
                    n228 = node-c288(w418) -> ()
                  }
                  frame Enabled {
                    n229 = while {
                      shift-right: [w461] -> _
                      shift-left: w451 -> [w455]
                      tunnel: w450 -> [w468]
                      tunnel: w452 -> [w466]
                      tunnel: w451 -> [w460]
                      tunnel: w449 -> [w454]
                      stop <- w465 continue-if-true
                      n230 = xnode ("Memory Read")("Address"=w455) -> ("Data"=w463:i16)  [unwired: 1 in, 1 out]
                      n231 = xnode ("Memory Read")("Address"=w455) -> ("Data"=w467:i16)  [unwired: 1 in, 1 out]
                      n232 = Equal?(x=w455, y=w468) -> (x = y?=w459:bool)
                      n233 = call "Loop Timer23"("Count(Ticks)"=w466) -> ()  [unwired: 1 out]
                      n234 = local read "Image Done?"() -> (w458:bool)
                      n235 = Increment(x=w455) -> (x+1=w469:u32)
                      n236 = And(x=w458, y=w459) -> (x .and. y?=w457:bool)
                      n237 = Select(t=w455, s=w459, f=w469) -> (s? t:f=w462:u32)
                      n238 = Less?(x=w462, y=u32 6) -> (x < y?=w456:bool)
                      n239 = local read "Start Waveforms"() -> (w465:bool)
                      n240 = xnode "FPGA I/O Node"("Connector0/AO6"=w463) -> ()  [unwired: 1 in, 1 out]
                      n241 = xnode "FPGA I/O Node"("Connector0/AO5"=w467) -> ()  [unwired: 1 in, 1 out]
                      n242 = Select(t=w460, s=w457, f=w462) -> (s? t:f=w461:u32)
                      n243 = Greater Or Equal?(x=w455, y=w454) -> (x >= y?=→"End Linear Ramp":bool)
                      n244 = local write "Frame Trigger"(w456) -> ()
                    }
                  }
                }
                n245 = while {
                  shift-right: [w492] -> _
                  shift-left: FALSE -> [w493]
                  shift-right: [w486] -> _
                  shift-left: w403 -> [w488]
                  tunnel: w405 -> [w487]
                  shift-right: [w470] -> _
                  shift-left: w401 -> [w483]
                  tunnel: w404 -> [w482]
                  shift-right: [w476] -> _
                  shift-left: w403 -> [w479]
                  tunnel: w402 -> [w475]
                  tunnel: w401 -> [w472]
                  tunnel: w399 -> [w471]
                  stop <- w494 continue-if-true
                  n246 = local read "End Linear Ramp"() -> (w492:bool)
                  n247 = Increment(x=w488) -> (x+1=w491:u8)
                  n248 = Greater?(x=w492, y=w493) -> (0:w490:bool)
                  n249 = Select(t=w491, s=w490, f=w488) -> (s? t:f=w485:u8)
                  n250 = Add(x=w482, y=w483) -> (x+y=w484:i16)
                  n251 = Increment(x=w479) -> (x+1=w480:u8)
                  n252 = Equal?(x=w485, y=w487) -> (x = y?=w481:bool)
                  n253 = Select(t=u8 0, s=w481, f=w485) -> (s? t:f=w486:u8)
                  n254 = Select(t=w480, s=w481, f=w479) -> (s? t:f=w477:u8)
                  n255 = Select(t=w484, s=w481, f=w483) -> (s? t:f=w478:i16)
                  n256 = call "Loop Timer21"("Count(Ticks)"=w471) -> ()  [unwired: 1 out]
                  n257 = Equal?(x=w477, y=w475) -> (x = y?=w474:bool)
                  n258 = local read "Start Waveforms"() -> (w494:bool)
                  n259 = Select(t=w472, s=w474, f=w478) -> (s? t:f=w470:i16)
                  n260 = xnode "FPGA I/O Node"("Connector0/AO3"=w470) -> ()  [unwired: 1 in, 1 out]
                  n261 = Select(t=u8 0, s=w474, f=w477) -> (s? t:f=w476:u8)
                }
              }
              frame 7 {
                w504 = u8 0
                n262 = node-c288() -> (w509:T4)  [unwired: 1 in]
                n263 = while {
                  shift-right: [w557] -> _
                  shift-left: w510 -> [w563]
                  tunnel: w497 -> [w564]
                  tunnel: w498 -> [w561]
                  tunnel: w510 -> [w560]
                  stop <- w559 continue-if-true
                  n264 = Increment(x=w563) -> (x+1=w565:u32)
                  n265 = Equal?(x=w563, y=w564) -> (x = y?=w558:bool)
                  n266 = xnode ("Memory Read")("Address"=w563) -> ("Data"=w562:i16)  [unwired: 1 in, 1 out]
                  n267 = Select(t=w560, s=w558, f=w565) -> (s? t:f=w557:u32)
                  n268 = call "Loop Timer4"("Count(Ticks)"=w561) -> ()  [unwired: 1 out]
                  n269 = Less?(x=w557, y=u32 20) -> (x < y?=w555:bool)
                  n270 = xnode "FPGA I/O Node"("TRIG0"=w555) -> ()  [unwired: 1 in, 1 out]
                  n271 = local read "Start Waveforms"() -> (w559:bool)
                  n272 = xnode "FPGA I/O Node"("Connector0/AO1"=w562) -> ()  [unwired: 1 in, 1 out]
                }
                n273 = while {
                  shift-right: [w511] -> _
                  shift-left: FALSE -> [w534]
                  shift-right: [w528] -> _
                  shift-left: w504 -> [w530]
                  tunnel: w506 -> [w529]
                  shift-right: [w512] -> _
                  shift-left: w502 -> [w525]
                  tunnel: w505 -> [w524]
                  shift-right: [w518] -> _
                  shift-left: w504 -> [w521]
                  tunnel: w503 -> [w517]
                  tunnel: w502 -> [w514]
                  tunnel: w499 -> [w513]
                  stop <- w535 continue-if-true
                  n274 = local read "End Linear Ramp"() -> (w511:bool)
                  n275 = Increment(x=w530) -> (x+1=w533:u8)
                  n276 = Greater?(x=w511, y=w534) -> (0:w532:bool)
                  n277 = Select(t=w533, s=w532, f=w530) -> (s? t:f=w527:u8)
                  n278 = Add(x=w524, y=w525) -> (x+y=w526:i16)
                  n279 = Increment(x=w521) -> (x+1=w522:u8)
                  n280 = Equal?(x=w527, y=w529) -> (x = y?=w523:bool)
                  n281 = Select(t=u8 0, s=w523, f=w527) -> (s? t:f=w528:u8)
                  n282 = Select(t=w522, s=w523, f=w521) -> (s? t:f=w519:u8)
                  n283 = Select(t=w526, s=w523, f=w525) -> (s? t:f=w520:i16)
                  n284 = call "Loop Timer17"("Count(Ticks)"=w513) -> ()  [unwired: 1 out]
                  n285 = Equal?(x=w519, y=w517) -> (x = y?=w516:bool)
                  n286 = local read "Start Waveforms"() -> (w535:bool)
                  n287 = Select(t=w514, s=w516, f=w520) -> (s? t:f=w512:i16)
                  n288 = xnode "FPGA I/O Node"("Connector0/AO3"=w512) -> ()  [unwired: 1 in, 1 out]
                  n289 = Select(t=u8 0, s=w516, f=w519) -> (s? t:f=w518:u8)
                }
                n290 = timed-loop {
                  timing: w509 -> [_]
                  timing-out: [_] -> w508
                  tunnel: w499 -> [w547]
                  tunnel: [w547] -> w500
                  tunnel: w496 -> [w548]
                  i -> [w550]
                  stop <- w549 stop-if-true
                  n291 = Equal?(x=w548, y=w550) -> (x = y?=w549:bool)
                }
                n292 = while {
                  shift-right: [w538] -> _
                  shift-left: w510 -> [w544]
                  tunnel: w495 -> [w545]
                  tunnel: w500 -> [w542]
                  tunnel: w510 -> [w541]
                  tunnel: w501 -> [w537]
                  stop <- w540 continue-if-true
                  n293 = Increment(x=w544) -> (x+1=w546:u32)
                  n294 = Equal?(x=w544, y=w545) -> (x = y?=w539:bool)
                  n295 = xnode ("Memory Read")("Address"=w544) -> ("Data"=w543:i16)  [unwired: 1 in, 1 out]
                  n296 = Select(t=w541, s=w539, f=w546) -> (s? t:f=w538:u32)
                  n297 = Greater?(x=w537, y=w538) -> (0:w536:bool)
                  n298 = local write "End Linear Ramp"(w536) -> ()
                  n299 = call "Loop Timer15"("Count(Ticks)"=w542) -> ()  [unwired: 1 out]
                  n300 = local read "Start Waveforms"() -> (w540:bool)
                  n301 = xnode "FPGA I/O Node"("Connector0/AO2"=w543) -> ()  [unwired: 1 in, 1 out]
                }
                n302 = node-c288(w508) -> ()
              }
            }
            n303 = case shown="3" w78 {
              frame 0, Default {
              }
              frame 3 {
                n304 = while {
                  stop <- w109 continue-if-true
                  n305 = local read "Start Waveforms"() -> (w109:bool)
                  n306 = xnode "FPGA I/O Node"("Connector0/AO1"="X Piezo Axis", "Connector0/AO2"="Y Piezo Axis", "Connector0/AO3"="Z Piezo Axis") -> ()  [unwired: 3 in, 3 out]
                }
              }
            }
            n307 = Index Array(array="Accums Per Line", index #1=0 ("index"), index #2=1 ("index"), index #3=2 ("index"), index #4=3 ("index")) -> (element #1=w87:u32, element #2=w86:u32, element #3=w85:u32, element #4=w84:u32)
            n308 = Compound Arithmetic op=ADD(w87, w86, w85, w84) -> (w94:u32)
            n309 = Multiply(x="Number of Lines", y=w94) -> (x*y=w95:u32)
            n310 = node-c288() -> (w97:T4)  [unwired: 1 in]
            n311 = timed-loop {
              timing: w97 -> [_]
              timing-out: [_] -> w96
              shift-right: [w134] -> _
              shift-left: w76 -> [w133]
              shift-right: [w131] -> _
              shift-left: _ -> [w125]
              shift-right: [w132] -> _
              shift-left: _ -> [w130]
              shift-right: [w119] -> _
              shift-left: u32 0 -> [w114]
              shift-right: [w127] -> _
              shift-left: w76 -> [w124]
              tunnel: w95 -> [w122]
              shift-right: [w111] -> _
              shift-left: w76 -> [w116]
              stop <- "Stop Sync Signal" continue-if-true
              n312 = Increment(x=w114) -> (x+1=w126:u32)
              n313 = Equal?(x=w114, y=w122) -> (x = y?=w115:bool)
              n314 = And(x=w125, y=w124) -> (x .and. y?=w129:bool)
              n315 = And(x=w124, y=w125) -> (x .and. y?=w123:bool)
              n316 = local read "Frame Trigger"() -> (w110:bool)
              n317 = case shown="True" w130 {
                tunnel: w129 -> [_ w135]
                frame False {
                }
                frame True {
                  n318 = xnode "FPGA I/O Node"("TRIG1"=w135) -> ()  [unwired: 1 in, 1 out]
                  "Laser Blank Trigger" <- w135
                }
              }
              n319 = Select(t=w126, s=w123, f=w114) -> (s? t:f=w121:u32)
              n320 = Equal?(x=w114, y=u32 10) -> (x = y?=w112:bool)
              n321 = Exclusive Or(1:w112, 2:w115) -> (0:w117:bool)
              n322 = Exclusive Or(1:w115, 2:w110) -> (0:w128:bool)
              n323 = xnode "FPGA I/O Node"() -> ("Connector1/DIO0"=w134:bool)  [unwired: 1 in, 1 out]
              n324 = Select(t=w115, s=w117, f=w116) -> (s? t:f=w111:bool)
              "Image Done?" <- w111
              n325 = Select(t=w110, s=w128, f=w124) -> (s? t:f=w127:bool)
              n326 = Select(t=u32 0, s=w115, f=w121) -> (s? t:f=w119:u32)
              n327 = Not Equal?(x=w134, y=w133) -> (x != y?=w132:bool)
              n328 = Greater?(x=w134, y=w133) -> (0:w131:bool)
            }
            n329 = node-c288(w96) -> ()
          }
        }
      }
    }
  }
  n330 = local read "Accums Per Line"() -> (w1:u32[])
  n331 = while {
    shift-right: [w614] -> _
    shift-left: u8 0 -> [w591]
    shift-right: [w615] -> _
    shift-left: w2 -> [w619]
    shift-right: [w613] -> _
    shift-left: u8 0 -> [w616]
    tunnel: "Sequences" -> [w612]
    shift-right: [w606] -> _
    shift-left: u32 0 -> [w607]
    tunnel: w1 -> [w593]
    shift-right: [w586] -> _
    shift-left: w2 -> [w585]
    stop <- FALSE stop-if-true
    n332 = local read "Laser Blank Trigger"() -> (w586:bool)
    n333 = To Long Integer(number=w591) -> (32bit integer=w590:i32)
    n334 = Add(x="Laser Delay (Ticks)", y="Laser On Time (Ticks)") -> (x+y=w573:u8)
    n335 = Index Array(array=w593, index=w590) -> (element=w592:u32)
    n336 = Increment(x=w607) -> (x+1=w608:u32)
    n337 = Equal?(x=w607, y=w592) -> (x = y?=w604:bool)
    n338 = Equal?(x=w616, y=w573) -> (x = y?=w605:bool)
    n339 = Greater?(x=w586, y=w585) -> (0:w584:bool)
    n340 = Select(t=w608, s=w605, f=w607) -> (s? t:f=w609:u32)
    n341 = Increment(x=w591) -> (x+1=w624:u8)
    n342 = Equal?(x=w591, y=w612) -> (x = y?=w621:bool)
    n343 = Exclusive Or(1:w605, 2:w584) -> (0:w620:bool)
    n344 = Select(t=u32 0, s=w604, f=w609) -> (s? t:f=w606:u32)
    n345 = Select(t=w624, s=w604, f=w591) -> (s? t:f=w623:u8)
    n346 = Increment(x=w616) -> (x+1=w618:u8)
    n347 = Select(t=w584, s=w620, f=w619) -> (s? t:f=w615:bool)
    n348 = Split Number(x="Laser States") -> (hi(x)=w601:u16, lo(x)=w602:u16)
    n349 = Select(t=u8 0, s=w621, f=w623) -> (s? t:f=w614:u8)
    n350 = Select(t=w618, s=w615, f=u8 0) -> (s? t:f=w613:u8)
    n351 = Split Number(x=w601) -> (hi(x)=w600:u8, lo(x)=w599:u8)
    n352 = Split Number(x=w602) -> (hi(x)=w598:u8, lo(x)=w597:u8)
    n353 = Greater?(x=w613, y="Laser Delay (Ticks)") -> (0:w588:bool)
    n354 = call "Loop Timer22"("Count(Ticks)"=u16 80) -> ()  [unwired: 1 out]
    n355 = case shown="0, Default" w614 {
      tunnel: w600 -> [w625 _ _ _]
      tunnel: w599 -> [_ w626 _ _]
      tunnel: w598 -> [_ _ w627 _]
      tunnel: w597 -> [_ _ _ w628]
      tunnel: [w625 w626 w627 w628] -> w596
      frame 0, Default {
      }
      frame 1 {
      }
      frame 2 {
      }
      frame 3 {
      }
    }
    n356 = Or(x="Blanking Off/Manual", y=w588) -> (x .or. y?=w589:bool)
    n357 = Select(t=w596, s=w589, f=u8 0) -> (s? t:f=w581:u8)
    n358 = Number To Boolean Array(number=w581) -> (Boolean array=w583:bool[])
    n359 = Index Array(array=w583, index #1=0 ("index"), index #2=1 ("index"), index #3=2 ("index"), index #4=3 ("index"), index #5=4 ("index")) -> (element #1=w577:bool, element #2=w576:bool, element #3=w571:bool, element #4=w575:bool, element #5=w566:bool)
    n360 = Select(t="590 Analog Voltage (I16)", s=w571, f=i16 0) -> (s? t:f=w569:i16)
    n361 = xnode "FPGA I/O Node"("Connector0/DIO0"=w577, "Connector1/DIO8"=w576, "Connector1/DIO9"=w575, "Connector1/DIO10"=w566) -> ()  [unwired: 4 in, 4 out]
    n362 = xnode "FPGA I/O Node"("Connector0/AO0"=w569) -> ()  [unwired: 1 in, 1 out]
  }
